vi "Calculate R and G (Four Terminal).vi"(8 "V-":i32, 9 "V+":i32, 10 "Current":i32, 11 "Lockin[ ]":dbl[](array[numeric])) -> (0 "G_4T (e2/h)":dbl, 1 "R_4T (h/e2)":dbl, 2 "G_4T (Siemens)":dbl, 3 "R_4T (ohms)":dbl)   [LabVIEW 2019, in "Transport.lvclass"]
uses:
  Transport.lvclass
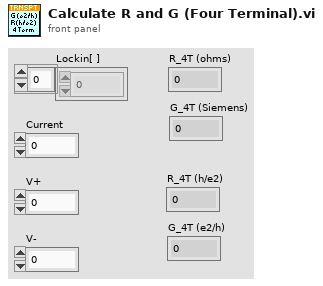
[diagram p1: front panel]
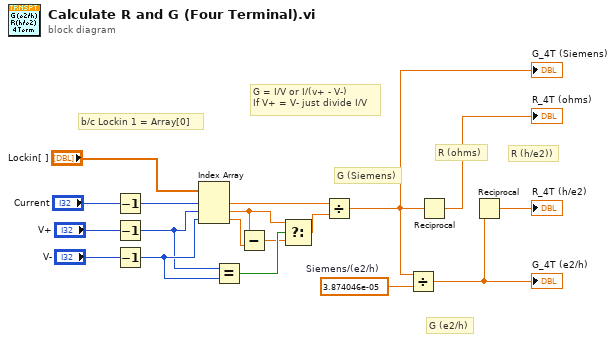
[diagram p0: block diagram]
diagram:
  w7 = 3.874046e-05  # Siemens/(e2/h)
  # "R (h/e2))"
  # "G (e2/h)"
  # "R (ohms)"
  # "G (Siemens)"
  # "b/c Lockin 1 = Array[0]"
  # "G = I/V or I/(v+ - V-)\nIf V+ = V- just divide I/V"
  n1 = Decrement(x="Current") -> (x-1=w8:i32)
  n2 = Decrement(x="V+") -> (x-1=w12:i32)
  n3 = Decrement(x="V-") -> (x-1=w13:i32)
  n4 = Index Array(array="Lockin[ ]", index #1=w8, index #2=w12, index #3=w13) -> (element #1=w6:dbl, element #2=w11:dbl, element #3=w9:dbl)
  n5 = Equal?(x=w12, y=w13) -> (x = y?=w14:bool)
  n6 = Subtract(x=w11, y=w9) -> (x-y=w10:dbl)
  n7 = Select(t=w11, s=w14, f=w10) -> (s? t:f=w5:dbl)
  n8 = Divide(x=w6, y=w5) -> (x/y=w1:dbl)
  "G_4T (Siemens)" <- w1
  n9 = Divide(x=w1, y=w7) -> (x/y=w4:dbl)
  "G_4T (e2/h)" <- w4
  n10 = Reciprocal(x=w1) -> (1/x=→"R_4T (ohms)":dbl)
  n11 = Reciprocal(x=w4) -> (1/x=→"R_4T (h/e2)":dbl)
